vi "Add Attribute Integer.vi"(8 "data":i32[](array[numeric]), 9 "Attribute name":string, 10 "loc_id":i32, 11 "error in (no error)":errorcluster) -> (0 "Error code":i32, 3 "error out":errorcluster)   [LabVIEW 2010]
uses:
  Release/hdf5_hldll.dll
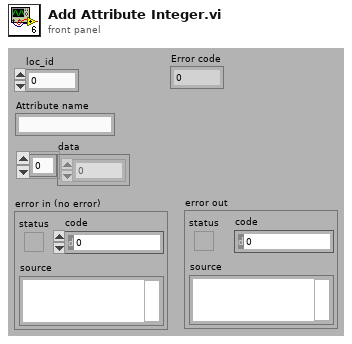
[diagram p1: front panel]
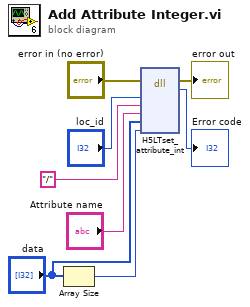
[diagram p0: block diagram]
diagram:
  n1 = Array Size(array="data") -> (size(s)=w2:i32)
  n2 = dll-call lib="Z:/users/alex/projects/HDF5Tools/Release/hdf5_hldll.dll" fn="H5LTset_attribute_int"(error in="error in (no error)", "loc_id"="loc_id", "obj_name"="/", "attr_name"="Attribute name", "data"="data", "size"=w2) -> (error out=→"error out":errorcluster, "error"=→"Error code":i32)  [unwired: 7 in, 1 out]
